vi "colors.vi"() -> ()   [LabVIEW 2021]
panel:
  in  "Colors":T1={"primary color"=6776679, "secondary color"=9671571, "accent color"=16741120, "background color"=16382457, "accent s color"=16668672}
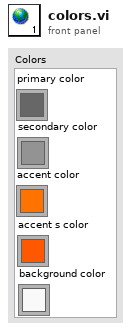
[diagram p1: front panel]
types:
  T1 = cluster{"primary color":u32, "secondary color":u32, "accent color":u32, "background color":u32, "accent s color":u32}
diagram:
